vi "Initialize Configuration Resource.vi"(8 "error in (no error)":errorcluster, 11 "TransientConfiguration in":refnum<class "TransientConfiguration.lvclass">) -> (0 "error out":errorcluster, 3 "TransientConfiguration out":refnum<class "TransientConfiguration.lvclass">)   [LabVIEW 2019, in "TransientConfiguration.lvclass"]
uses:
  <vilib>/gpm_packages/@cs/Configuration/Source/TransientConfiguration/TransientConfiguration.lvclass
  <vilib>/gpm_packages/@cs/Configuration/Source/TransientConfiguration/TransientConfiguration.lvclass/TransientConfiguration.ctl
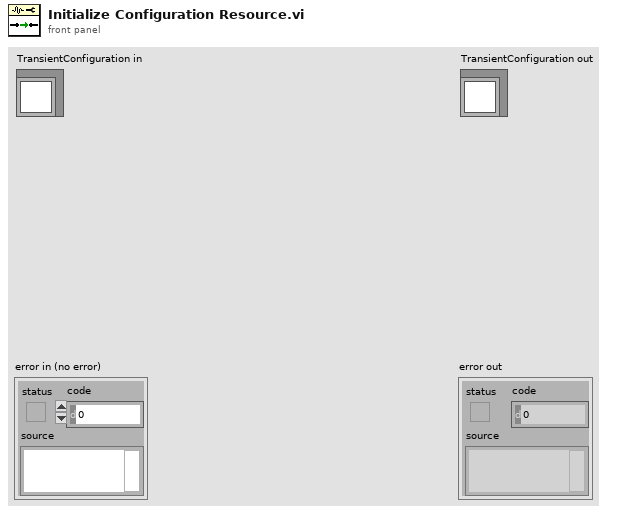
[diagram p1: front panel]
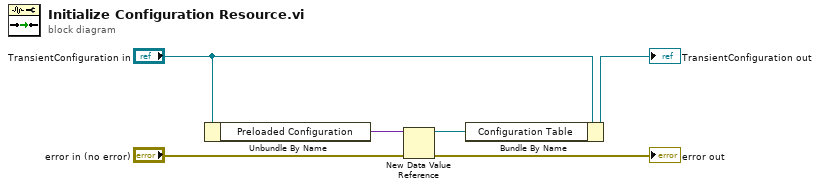
[diagram p0: block diagram]
diagram:
  n1 = Unbundle By Name("TransientConfiguration in") -> ("Preloaded Configuration"=w1:variant)
  n2 = New Data Value Reference(data value=w1, error in="error in (no error)") -> (data value reference=w3:refnum<data-value>, error out=→"error out":errorcluster)
  n3 = Bundle By Name(cluster="TransientConfiguration in", "Configuration Table"=w3) -> (→"TransientConfiguration out":refnum<class "TransientConfiguration.lvclass">)
